vi "PicoScope2000aGetRapidBlockBulk.vi"(0 "error in":errorcluster, 1 "enabled array":i16[](array[numeric]), 7 "handle in":i16, 9 "Device Info":T2, 11 "Rapid Block Acquisition Settings":T1 {"Down Sample Ratio" min=1 step=1; "Down-Sample Mode" items=["None", "Aggregate", "Decimate", "Average"]}) -> (2 "Channel A Buffer":i16[][](array[numeric]), 3 "Channel B Buffer":i16[][](array[numeric]), 4 "error out":errorcluster, 6 "handle out":i16, 10 "Port 0":i16[][](array[numeric]), 12 "Num samples":u32, 13 "Channel C Buffer":i16[][](array[numeric]), 14 "Channel D Buffer":i16[][](array[numeric]), 15 "Port 1":i16[][](array[numeric]))   [LabVIEW 2009]
doc: "This VI gets a set of blocks captured using rapid block mode. It outputs two-dimensional arrays for each channel that contain data from all the requested captures.\n'Enabled array' must be connected, it contains elements related to enabled channel(s).\nNormally connected from PicoScope2000aSettings.vi\nEach 16-bit element relates to channels in order of A-D, Port0, Port1.\nWhere '0' represents a disabled channel and '1' represents an enabled channel."
uses:
  ps2000a.dll
panel:
  out "nMaxSamples":i32
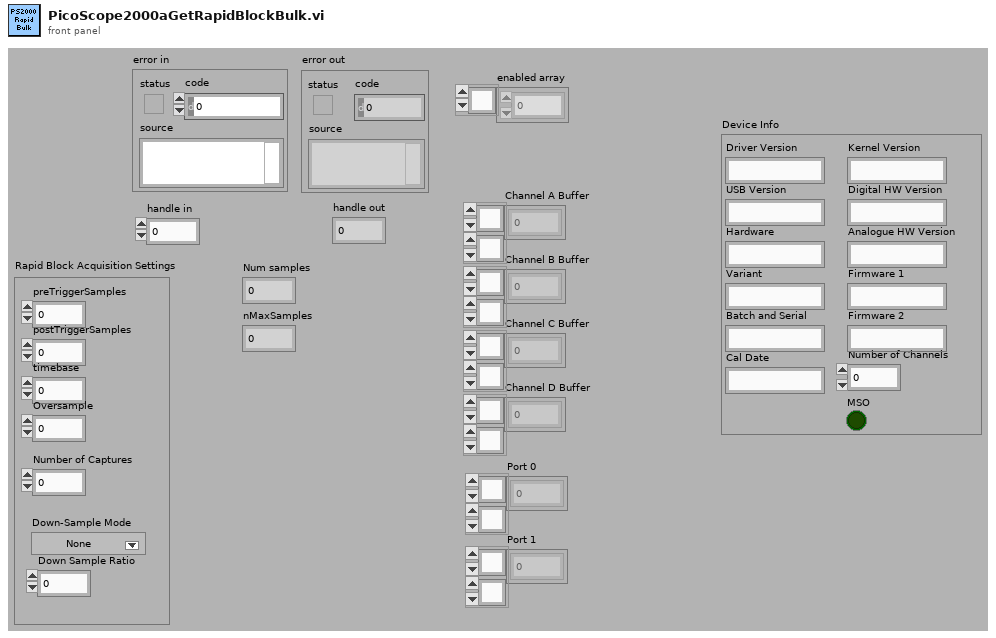
[diagram p1: front panel]
types:
  T1 = cluster{"preTriggerSamples":u32, "postTriggerSamples":u32, "timebase":u32, "Down-Sample Mode":i32, "Down Sample Ratio":u32, "Oversample":i16, "Number of Captures":u32}
  T2 = cluster{"Driver Version":string, "USB Version":string, "Hardware":string, "Variant":string, "Batch and Serial":string, "Cal Date":string, "Kernel Version":string, "Digital HW Version":string, "Analogue HW Version":string, "Firmware 1":string, "Firmware 2":string, "MSO":bool, "Number of Channels":i16}
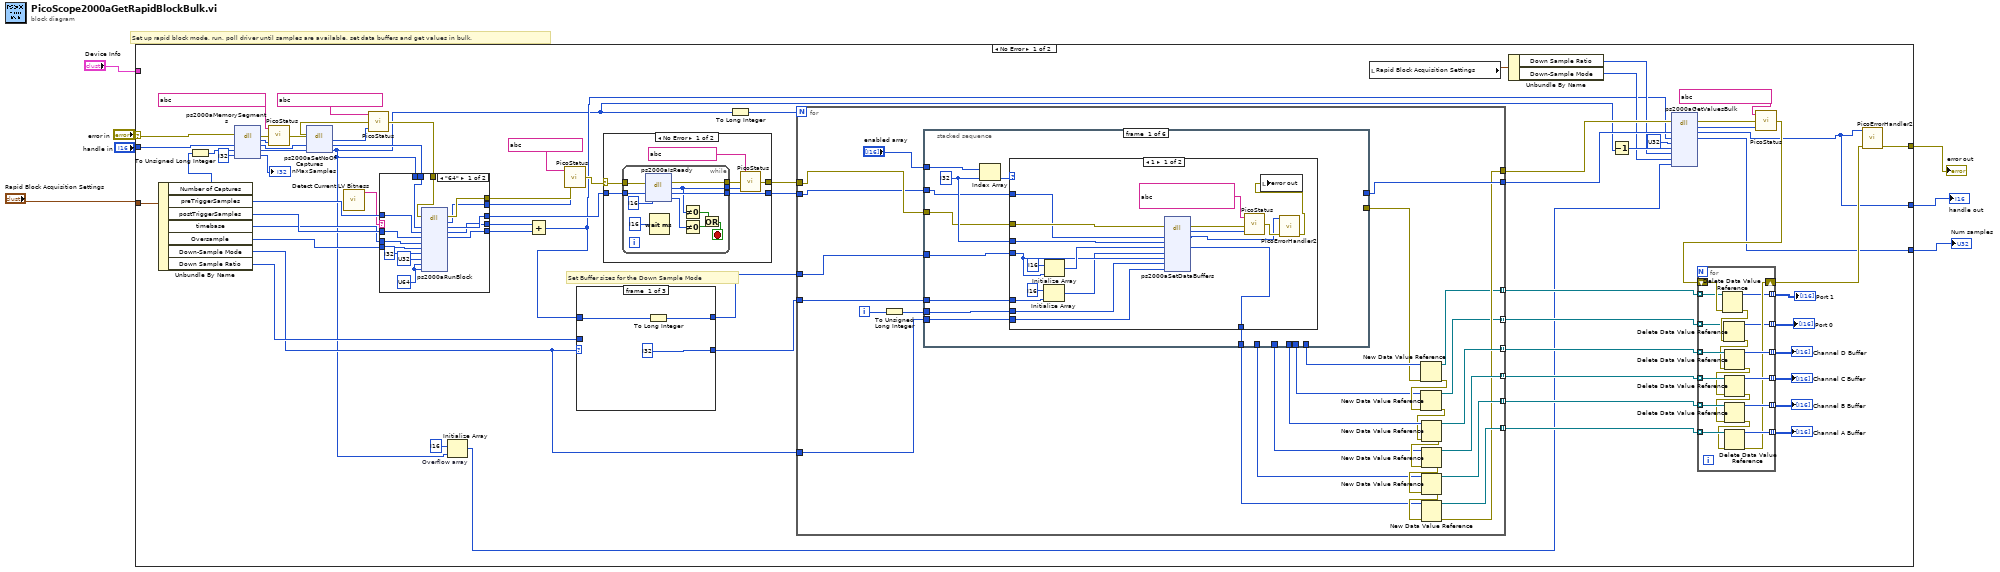
[diagram p0: block diagram]
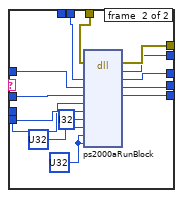
[diagram p2: hidden frame]
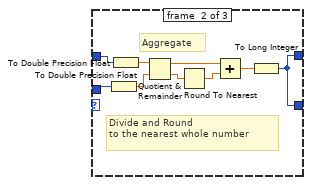
[diagram p3: hidden frame]
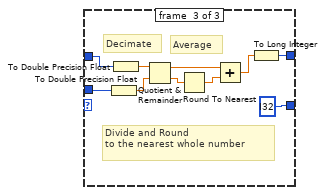
[diagram p4: hidden frame]
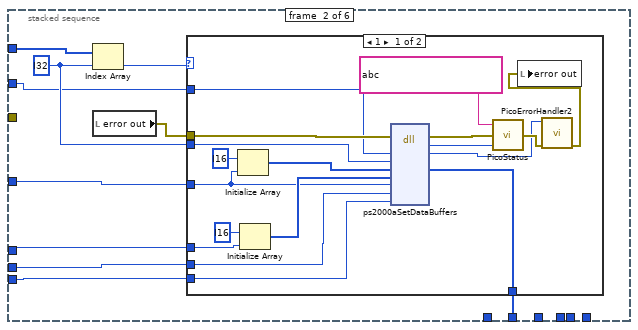
[diagram p6: hidden frame]
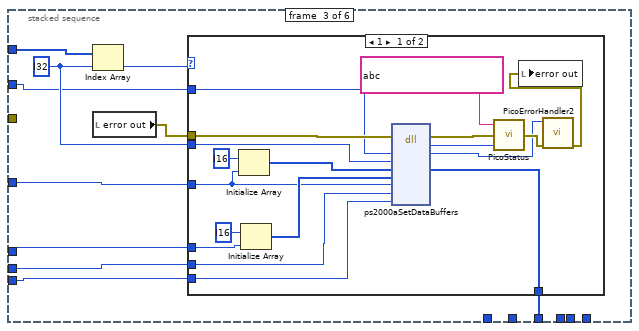
[diagram p8: hidden frame]
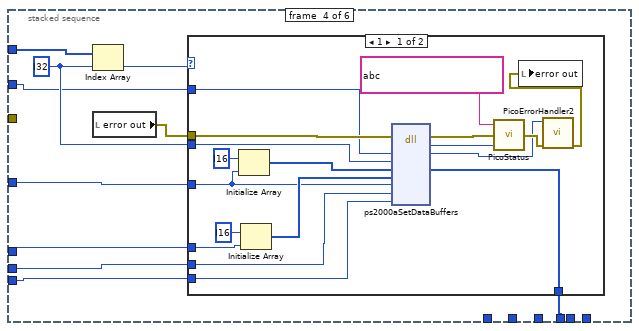
[diagram p10: hidden frame]
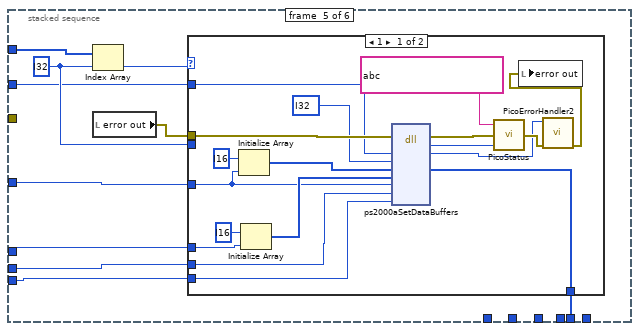
[diagram p12: hidden frame]
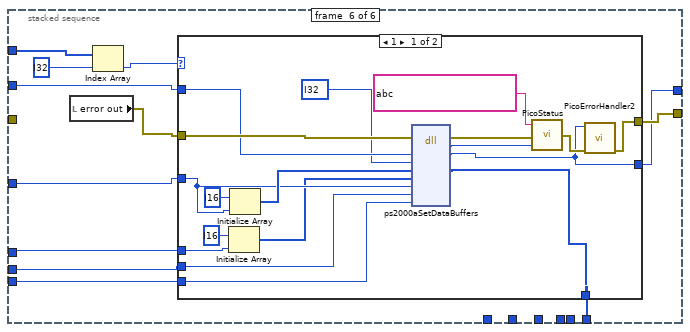
[diagram p14: hidden frame]
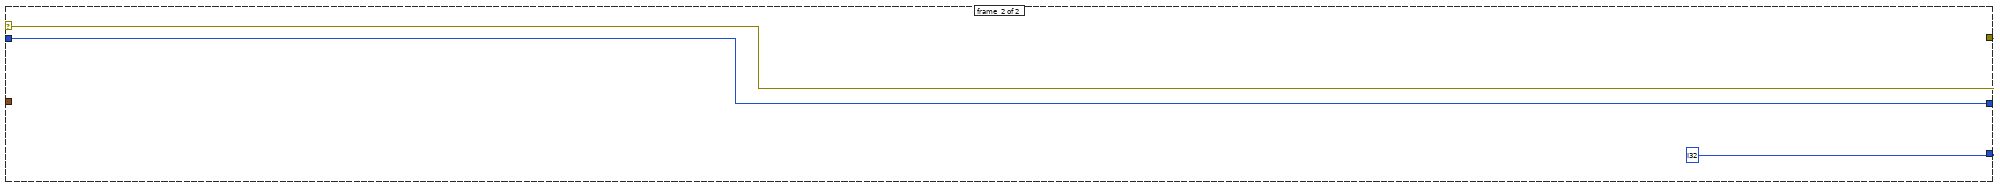
[diagram p17: hidden frame]
diagram:
  # "Set up rapid block mode, run, poll driver until samples are available, set data buffers and get values in bulk."
  n1 = case shown="No Error" "error in" {
    selector: "error in" -> [w73 w365]
    tunnel: "handle in" -> [w72 w367]
    tunnel: [w16 w367] -> w5
    tunnel: [w37 i32 ?] -> w4
    tunnel: "Device Info" -> [_ _]
    tunnel: "Rapid Block Acquisition Settings" -> [w60 _]
    tunnel: [w42 w365] -> w1
    frame #0 {
      # "Set Buffer sizes for the Down Sample Mode"
      n2 = Unbundle By Name(w60) -> ("Number of Captures"=w53:u32, "preTriggerSamples"=w15:u32, "postTriggerSamples"=w14:u32, "timebase"=w13:u32, "Oversample"=w12:i16, "Down-Sample Mode"=w18:i32, "Down Sample Ratio"=w19:u32)
      n3 = To Unsigned Long Integer(number=w53) -> (unsigned 32bit integer=w54:u32)
      n4 = dll-call lib="ps2000a.dll" fn="ps2000aMemorySegments" ("ps3000.dll:_ps3000_open_unit@0")(error in=w73, "handle"=w72, "nSegments"=w54, "nMaxSamples"=i32 ?) -> (error out=w70:errorcluster, "PICO_STATUS"=w71:i32, "handle"=w66:i16, "nSegments"=w67:u32, "nMaxSamples"=→"nMaxSamples":i32)  [unwired: 2 in, 1 out]
      n5 = call "PicoStatus.vi"("PICO STATUS"=w71, "error in"=w70, "source"=string ?) -> ("error out"=w65:errorcluster)
      n6 = dll-call lib="ps2000a.dll" fn="ps2000aSetNoOfCaptures" ("ps3000.dll:_ps3000_open_unit@0")(error in=w65, "handle"=w66, "nCaptures"=w67) -> (error out=w63:errorcluster, "PICO_STATUS"=w64:i32, "handle"=w58:i16, "nCaptures"=w10:u32)  [unwired: 2 in, 1 out]
      n7 = call "Detect Current LV Bitness.vi"() -> ("bitness"=w11:string)  [unwired: 11 in]
      n8 = call "PicoStatus.vi"("PICO STATUS"=w64, "error in"=w63, "source"=string ?) -> ("error out"=w59:errorcluster)
      n9 = case shown="\"64\"" w11 {
        tunnel: w59 -> [w89 w103]
        tunnel: w58 -> [w76 w102]
        tunnel: [w84 w101] -> w57
        tunnel: [w83 w100] -> w56
        tunnel: [w82 w99] -> w55
        tunnel: w15 -> [w88 w98]
        tunnel: w14 -> [w87 w97]
        tunnel: w13 -> [w86 w96]
        tunnel: w12 -> [w85 w95]
        tunnel: w10 -> [_ _]
        tunnel: [w81 w92] -> w9
        tunnel: [w80 w91] -> w8
        frame #0 {
          w77 = u64 ? ("pParameter")
          n10 = dll-call lib="ps2000a.dll" fn="ps2000aRunBlock" ("ps3000.dll:_ps3000_open_unit@0")(error in=w89, "handle"=w76, "preTriggerSamples"=w88, "postTriggerSamples"=w87, "timebase"=w86, "oversample"=w85, "timeindisposed"=i32 ?, "segmentIndex"=u32 ?, "lpReady"=w77, "pParameter"=w77) -> (error out=w84:errorcluster, "PICO_STATUS"=w83:i32, "handle"=w82:i16, "preTriggerSamples"=w81:u32, "postTriggerSamples"=w80:u32)  [unwired: 8 in, 1 out]
        }
        frame #1 {
          w90 = u32 ? ("pParameter")
          n11 = dll-call lib="ps2000a.dll" fn="ps2000aRunBlock" ("ps3000.dll:_ps3000_open_unit@0")(error in=w103, "handle"=w102, "preTriggerSamples"=w98, "postTriggerSamples"=w97, "timebase"=w96, "oversample"=w95, "timeindisposed"=i32 ?, "segmentIndex"=u32 ?, "lpReady"=w90, "pParameter"=w90) -> (error out=w101:errorcluster, "PICO_STATUS"=w100:i32, "handle"=w99:i16, "preTriggerSamples"=w92:u32, "postTriggerSamples"=w91:u32)  [unwired: 8 in, 1 out]
        }
      }
      n12 = Initialize Array "Overflow array"(i16 ? ("element"), w10) -> (w27:i16[])
      n13 = Add(x=w9, y=w8) -> (x+y=w20:u32)
      n14 = call "PicoStatus.vi"("PICO STATUS"=w56, "error in"=w57, "source"=string ?) -> ("error out"=w75:errorcluster)
      n15 = case shown="Default" w18 {
        tunnel: w19 -> [_ w107 w117]
        tunnel: w20 -> [w106 w108 w119]
        tunnel: [w105 w115 w125] -> w22
        tunnel: [i32 ? w115 i32 ?] -> w21
        frame #0 {
          n16 = To Long Integer(number=w106) -> (32bit integer=w105:i32)
        }
        frame #1 {
          # "Divide and Round\nto the nearest whole number"
          # "Aggregate"
          n17 = To Double Precision Float(number=w107) -> (double precision float=w110:dbl)
          n18 = To Double Precision Float(number=w108) -> (double precision float=w111:dbl)
          n19 = Quotient & Remainder(x=w111, y=w110) -> (x-y*floor(x/y)=w112:dbl, floor(x/y)=w114:dbl)
          n20 = Round To Nearest(number=w114) -> (nearest integer value=w113:dbl)
          n21 = Add(x=w112, y=w113) -> (x+y=w109:dbl)
          n22 = To Long Integer(number=w109) -> (32bit integer=w115:i32)
        }
        frame #2 {
          # "Divide and Round\nto the nearest whole number"
          # "Average"
          # "Decimate"
          n23 = To Double Precision Float(number=w117) -> (double precision float=w116:dbl)
          n24 = To Double Precision Float(number=w119) -> (double precision float=w118:dbl)
          n25 = Quotient & Remainder(x=w118, y=w116) -> (x-y*floor(x/y)=w121:dbl, floor(x/y)=w123:dbl)
          n26 = Round To Nearest(number=w123) -> (nearest integer value=w122:dbl)
          n27 = Add(x=w121, y=w122) -> (x+y=w120:dbl)
          n28 = To Long Integer(number=w120) -> (32bit integer=w125:i32)
        }
      }
      n29 = case shown="No Error" w75 {
        selector: w75 -> [w349 w363]
        tunnel: w55 -> [w351 w364]
        tunnel: [w350 w364] -> w50
        tunnel: [w348 w363] -> w51
        frame #0 {
          n30 = while {
            tunnel: [w353] -> w350
            tunnel: w351 -> [w357]
            tunnel: [w352] -> w346
            tunnel: w349 -> [w358]
            tunnel: [w355] -> w347
            stop <- w362 stop-if-true
            n31 = dll-call lib="ps2000a.dll" fn="ps2000aIsReady" ("ps3000.dll:_ps3000_open_unit@0")(error in=w358, "handle"=w357, "ready"=i16 ?) -> (error out=w355:errorcluster, "status"=w352:i32, "handle"=w353:i16, "ready"=w354:i16)  [unwired: 2 in, 1 out]
            n32 = Wait (ms)(milliseconds to wait=i16 ? ("ready")) -> ()  [unwired: 1 out]
            n33 = Not Equal To 0?(x=w352) -> (x != 0?=w360:bool)
            n34 = Not Equal To 0?(x=w354) -> (x != 0?=w361:bool)
            n35 = Or(x=w360, y=w361) -> (x .or. y?=w362:bool)
          }
          n36 = call "PicoStatus.vi"("PICO STATUS"=w346, "error in"=w347, "source"=string ?) -> ("error out"=w348:errorcluster)
        }
        frame #1 {
        }
      }
      n37 = To Long Integer(number=w10) -> (32bit integer=w49:i32)
      n38 = for {
        N: w49 -> [_]
        tunnel: w50 -> [w162]
        tunnel: w51 -> [w163]
        tunnel: [w155] -> w36
        tunnel: [w169] -> w32 mode=indexing
        tunnel: [w168] -> w31 mode=indexing
        tunnel: [w167] -> w30 mode=indexing
        tunnel: [w166] -> w29 mode=indexing
        tunnel: [w161] -> w35
        tunnel: w22 -> [w164]
        tunnel: [w150] -> w33 mode=indexing
        tunnel: [w149] -> w34 mode=indexing
        tunnel: w21 -> [w146]
        tunnel: w18 -> [w145]
        i -> [w148]
        n39 = To Unsigned Long Integer(number=w148) -> (unsigned 32bit integer=w147:u32)
        n40 = stacked-sequence {
          tunnel: "enabled array" -> [w181 w209 w237 w265 w293 w323]
          tunnel: w163 -> [w179 _ _ _ _ _]
          tunnel: w162 -> [w178 w207 w235 w263 w285 w318]
          tunnel: w164 -> [w175 w206 w234 w262 w292 w315]
          tunnel: [w177 _ _ _ _ _] -> w160
          tunnel: [_ _ _ _ _ w322] -> w152
          tunnel: [_ _ _ _ _ w321] -> w161
          tunnel: w147 -> [w176 w205 w233 w261 w291 w317]
          tunnel: [_ w204 _ _ _ _] -> w159
          tunnel: [_ _ w229 _ _ _] -> w158
          tunnel: [_ _ _ w257 _ _] -> w157
          tunnel: [_ _ _ _ w287 _] -> w154
          tunnel: [_ _ _ _ _ w314] -> w153
          tunnel: w146 -> [w174 w202 w231 w259 w289 w316]
          tunnel: w145 -> [w173 w201 w230 w258 w288 w313]
          frame #0 {
            w182 = i32 ? ("dimension size")
            n41 = Index Array(array=w181, index=w182) -> (element=w180:i16)
            n42 = case shown="1" w180 {
              tunnel: w182 -> [w194 _]
              tunnel: w179 -> [w196 _]
              tunnel: w178 -> [w195 _]
              tunnel: w175 -> [w192 _]
              tunnel: [w187 _] -> w177
              tunnel: w176 -> [w191 _]
              tunnel: w174 -> [w186 _]
              tunnel: w173 -> [w183 _]
              frame #0 {
                n43 = Initialize Array(i16 ? ("element"), w186) -> (w185:i16[])
                n44 = Initialize Array(i16 ? ("element"), w192) -> (w193:i16[])
                n45 = dll-call lib="ps2000a.dll" fn="ps2000aSetDataBuffers" ("ps3000.dll:_ps3000_open_unit@0")(error in=w196, "handle"=w195, "channel"=w194, "bufferMax"=w193, "bufferMin"=w185, "bufferLth"=w192, "segmentIndex"=w191, "downSampleRatioMode"=w183) -> (error out=w190:errorcluster, "PICO_STATUS"=w189:i32, "handle"=w188:i16, "bufferMax"=w187:i16[])  [unwired: 7 in, 1 out]
                n46 = call "PicoStatus.vi"("PICO STATUS"=w189, "error in"=w190, "source"=string ?) -> ("error out"=w199:errorcluster)
                n47 = call "PicoErrorHandler2.vi"("error in (no error)"=w199, "handle In"=w188) -> ("error out"=w198:errorcluster)  [unwired: 9 in]
                n48 = local write "error out"(w198) -> ()
              }
              frame #1 {
              }
            }
          }
          frame #1 {
            w210 = i32 ? ("dimension size")
            n49 = Index Array(array=w209, index=w210) -> (element=w208:i16)
            n50 = local read "error out"() -> (w203:errorcluster)
            n51 = case shown="1" w208 {
              tunnel: w210 -> [w214 _]
              tunnel: w203 -> [w219 _]
              tunnel: w207 -> [w211 _]
              tunnel: w206 -> [w217 _]
              tunnel: [w213 _] -> w204
              tunnel: w205 -> [w218 _]
              tunnel: w202 -> [w216 _]
              tunnel: w201 -> [w212 _]
              frame #0 {
                n52 = Initialize Array(i16 ? ("element"), w217) -> (w226:i16[])
                n53 = Initialize Array(i16 ? ("element"), w216) -> (w225:i16[])
                n54 = dll-call lib="ps2000a.dll" fn="ps2000aSetDataBuffers" ("ps3000.dll:_ps3000_open_unit@0")(error in=w219, "handle"=w211, "channel"=w214, "bufferMax"=w226, "bufferMin"=w225, "bufferLth"=w217, "segmentIndex"=w218, "downSampleRatioMode"=w212) -> (error out=w223:errorcluster, "PICO_STATUS"=w221:i32, "handle"=w220:i16, "bufferMax"=w213:i16[])  [unwired: 7 in, 1 out]
                n55 = call "PicoStatus.vi"("PICO STATUS"=w221, "error in"=w223, "source"=string ?) -> ("error out"=w227:errorcluster)
                n56 = call "PicoErrorHandler2.vi"("error in (no error)"=w227, "handle In"=w220) -> ("error out"=w228:errorcluster)  [unwired: 9 in]
                n57 = local write "error out"(w228) -> ()
              }
              frame #1 {
              }
            }
          }
          frame #2 {
            w238 = i32 ? ("dimension size")
            n58 = Index Array(array=w237, index=w238) -> (element=w236:i16)
            n59 = local read "error out"() -> (w232:errorcluster)
            n60 = case shown="1" w236 {
              tunnel: w238 -> [w242 _]
              tunnel: w232 -> [w247 _]
              tunnel: w235 -> [w239 _]
              tunnel: w234 -> [w245 _]
              tunnel: [w241 _] -> w229
              tunnel: w233 -> [w246 _]
              tunnel: w231 -> [w244 _]
              tunnel: w230 -> [w240 _]
              frame #0 {
                n61 = Initialize Array(i16 ? ("element"), w245) -> (w254:i16[])
                n62 = Initialize Array(i16 ? ("element"), w244) -> (w253:i16[])
                n63 = dll-call lib="ps2000a.dll" fn="ps2000aSetDataBuffers" ("ps3000.dll:_ps3000_open_unit@0")(error in=w247, "handle"=w239, "channel"=w242, "bufferMax"=w254, "bufferMin"=w253, "bufferLth"=w245, "segmentIndex"=w246, "downSampleRatioMode"=w240) -> (error out=w251:errorcluster, "PICO_STATUS"=w249:i32, "handle"=w248:i16, "bufferMax"=w241:i16[])  [unwired: 7 in, 1 out]
                n64 = call "PicoStatus.vi"("PICO STATUS"=w249, "error in"=w251, "source"=string ?) -> ("error out"=w255:errorcluster)
                n65 = call "PicoErrorHandler2.vi"("error in (no error)"=w255, "handle In"=w248) -> ("error out"=w256:errorcluster)  [unwired: 9 in]
                n66 = local write "error out"(w256) -> ()
              }
              frame #1 {
              }
            }
          }
          frame #3 {
            w266 = i32 ? ("dimension size")
            n67 = Index Array(array=w265, index=w266) -> (element=w264:i16)
            n68 = local read "error out"() -> (w260:errorcluster)
            n69 = case shown="1" w264 {
              tunnel: w266 -> [w270 _]
              tunnel: w260 -> [w275 _]
              tunnel: w263 -> [w267 _]
              tunnel: w262 -> [w273 _]
              tunnel: [w269 _] -> w257
              tunnel: w261 -> [w274 _]
              tunnel: w259 -> [w272 _]
              tunnel: w258 -> [w268 _]
              frame #0 {
                n70 = Initialize Array(i16 ? ("element"), w273) -> (w282:i16[])
                n71 = Initialize Array(i16 ? ("element"), w272) -> (w281:i16[])
                n72 = dll-call lib="ps2000a.dll" fn="ps2000aSetDataBuffers" ("ps3000.dll:_ps3000_open_unit@0")(error in=w275, "handle"=w267, "channel"=w270, "bufferMax"=w282, "bufferMin"=w281, "bufferLth"=w273, "segmentIndex"=w274, "downSampleRatioMode"=w268) -> (error out=w279:errorcluster, "PICO_STATUS"=w277:i32, "handle"=w276:i16, "bufferMax"=w269:i16[])  [unwired: 7 in, 1 out]
                n73 = call "PicoStatus.vi"("PICO STATUS"=w277, "error in"=w279, "source"=string ?) -> ("error out"=w283:errorcluster)
                n74 = call "PicoErrorHandler2.vi"("error in (no error)"=w283, "handle In"=w276) -> ("error out"=w284:errorcluster)  [unwired: 9 in]
                n75 = local write "error out"(w284) -> ()
              }
              frame #1 {
              }
            }
          }
          frame #4 {
            w294 = i32 ? ("dimension size")
            n76 = Index Array(array=w293, index=w294) -> (element=w286:i16)
            n77 = local read "error out"() -> (w290:errorcluster)
            n78 = case shown="1" w286 {
              tunnel: w294 -> [_ _]
              tunnel: w290 -> [w303 _]
              tunnel: w292 -> [w301 _]
              tunnel: [w298 _] -> w287
              tunnel: w291 -> [w302 _]
              tunnel: w289 -> [w300 _]
              tunnel: w288 -> [w297 _]
              tunnel: w285 -> [w295 _]
              frame #0 {
                n79 = Initialize Array(i16 ? ("element"), w301) -> (w310:i16[])
                n80 = Initialize Array(i16 ? ("element"), w300) -> (w309:i16[])
                n81 = dll-call lib="ps2000a.dll" fn="ps2000aSetDataBuffers" ("ps3000.dll:_ps3000_open_unit@0")(error in=w303, "handle"=w295, "channel"=i32 ?, "bufferMax"=w310, "bufferMin"=w309, "bufferLth"=w301, "segmentIndex"=w302, "downSampleRatioMode"=w297) -> (error out=w307:errorcluster, "PICO_STATUS"=w305:i32, "handle"=w304:i16, "bufferMax"=w298:i16[])  [unwired: 7 in, 1 out]
                n82 = call "PicoStatus.vi"("PICO STATUS"=w305, "error in"=w307, "source"=string ?) -> ("error out"=w311:errorcluster)
                n83 = call "PicoErrorHandler2.vi"("error in (no error)"=w311, "handle In"=w304) -> ("error out"=w312:errorcluster)  [unwired: 9 in]
                n84 = local write "error out"(w312) -> ()
              }
              frame #1 {
              }
            }
          }
          frame #5 {
            n85 = local read "error out"() -> (w320:errorcluster)
            n86 = Index Array(array=w323, index=i32 ? ("dimension size")) -> (element=w319:i16)
            n87 = case shown="1" w319 {
              tunnel: w320 -> [w339 w344]
              tunnel: w318 -> [w338 w343]
              tunnel: w315 -> [w336 _]
              tunnel: [w332 _] -> w314
              tunnel: w317 -> [w335 _]
              tunnel: w316 -> [w331 _]
              tunnel: [w328 w344] -> w322
              tunnel: [w327 w343] -> w321
              tunnel: w313 -> [w325 _]
              frame #0 {
                n88 = Initialize Array(i16 ? ("element"), w331) -> (w330:i16[])
                n89 = Initialize Array(i16 ? ("element"), w336) -> (w337:i16[])
                n90 = dll-call lib="ps2000a.dll" fn="ps2000aSetDataBuffers" ("ps3000.dll:_ps3000_open_unit@0")(error in=w339, "handle"=w338, "channel"=i32 ?, "bufferMax"=w337, "bufferMin"=w330, "bufferLth"=w336, "segmentIndex"=w335, "downSampleRatioMode"=w325) -> (error out=w334:errorcluster, "PICO_STATUS"=w333:i32, "handle"=w327:i16, "bufferMax"=w332:i16[])  [unwired: 7 in, 1 out]
                n91 = call "PicoStatus.vi"("PICO STATUS"=w333, "error in"=w334, "source"=string ?) -> ("error out"=w341:errorcluster)
                n92 = call "PicoErrorHandler2.vi"("error in (no error)"=w341, "handle In"=w327) -> ("error out"=w328:errorcluster)  [unwired: 9 in]
              }
              frame #1 {
              }
            }
          }
        }
        n93 = New Data Value Reference(data value=w153, error in=w152) -> (data value reference=w149:refnum<data-value>, error out=w156:errorcluster)
        n94 = New Data Value Reference(data value=w154, error in=w156) -> (data value reference=w150:refnum<data-value>, error out=w151:errorcluster)
        n95 = New Data Value Reference(data value=w157, error in=w151) -> (data value reference=w169:refnum<data-value>, error out=w172:errorcluster)
        n96 = New Data Value Reference(data value=w158, error in=w172) -> (data value reference=w168:refnum<data-value>, error out=w171:errorcluster)
        n97 = New Data Value Reference(data value=w159, error in=w171) -> (data value reference=w167:refnum<data-value>, error out=w170:errorcluster)
        n98 = New Data Value Reference(data value=w160, error in=w170) -> (data value reference=w166:refnum<data-value>, error out=w155:errorcluster)
      }
      n99 = local read "Rapid Block Acquisition Settings"() -> (w26:T1)
      n100 = Unbundle By Name(w26) -> ("Down Sample Ratio"=w25:u32, "Down-Sample Mode"=w24:i32)
      n101 = Decrement(x=w10) -> (x-1=w28:u32)
      n102 = dll-call lib="ps2000a.dll" fn="ps2000aGetValuesBulk" ("ps3000.dll:_ps3000_open_unit@0")(error in=w36, "handle"=w35, "noOfSamples"=w20, "fromSegmentIndex"=u32 ?, "toSegmentIndex"=w28, "downSampleRatio"=w25, "downSampleRatioMode"=w24, "overflow"=w27) -> (error out=w39:errorcluster, "PICO_STATUS"=w17:i32, "handle"=w16:i16, "noOfSamples"=w37:u32)  [unwired: 7 in, 1 out]
      n103 = call "PicoStatus.vi"("PICO STATUS"=w17, "error in"=w39, "source"=string ?) -> ("error out"=w40:errorcluster)
      n104 = for {
        tunnel: w29 -> [w144] mode=indexing
        tunnel: [w143] -> w45 mode=indexing
        shift-right: [w133] -> w41
        shift-left: w40 -> [w132]
        tunnel: w30 -> [w142] mode=indexing
        tunnel: w32 -> [w141] mode=indexing
        tunnel: w31 -> [w140] mode=indexing
        tunnel: [w136] -> w48 mode=indexing
        tunnel: [w135] -> w47 mode=indexing
        tunnel: [w134] -> w46 mode=indexing
        tunnel: w33 -> [w129] mode=indexing
        tunnel: w34 -> [w128] mode=indexing
        tunnel: [w127] -> w44 mode=indexing
        tunnel: [w126] -> w43 mode=indexing
        n105 = Delete Data Value Reference(data value reference=w128, error in=w132) -> (data value=w126:i16[], error out=w131:errorcluster)
        n106 = Delete Data Value Reference(data value reference=w129, error in=w131) -> (data value=w127:i16[], error out=w130:errorcluster)
        n107 = Delete Data Value Reference(data value reference=w141, error in=w130) -> (data value=w136:i16[], error out=w139:errorcluster)
        n108 = Delete Data Value Reference(data value reference=w140, error in=w139) -> (data value=w135:i16[], error out=w138:errorcluster)
        n109 = Delete Data Value Reference(data value reference=w142, error in=w138) -> (data value=w134:i16[], error out=w137:errorcluster)
        n110 = Delete Data Value Reference(data value reference=w144, error in=w137) -> (data value=w143:i16[], error out=w133:errorcluster)
      }
      "Channel D Buffer" <- w48
      "Channel C Buffer" <- w47
      "Channel B Buffer" <- w46
      "Channel A Buffer" <- w45
      "Port 0" <- w44
      "Port 1" <- w43
      n111 = call "PicoErrorHandler2.vi"("error in (no error)"=w41, "handle In"=w16) -> ("error out"=w42:errorcluster)  [unwired: 9 in]
    }
    frame #1 {
    }
  }
  "handle out" <- w5
  "Num samples" <- w4
  "error out" <- w1
